vi "recondense_Splitt_Cluster.vi"(0 "Recondense-Monitor":T3 {"He3-Pot Heater %" format="%#_4g"; "He3-Pot Setpoint" format="%#_4g"; "Sorb Heater %" format="%#_4g"; "Sorb Setpoint" format="%#_4g"; "He3 Temp2" format="%#_4g"; "He3 Temp 1" format="%#_4g"; "1K Temp" format="%#_4g"; "Sorb Temp" format="%#_4g"}) -> (1 "Recondense-Status":T2, 2 "Recondense-Control":T1)   [LabVIEW 2019]
uses:
  Brosowski/BorowskiMonitor.ctl
  Brosowski/Borowski-Status-Cluster.ctl
  Brosowski/Borowski-Control-Cluster.ctl
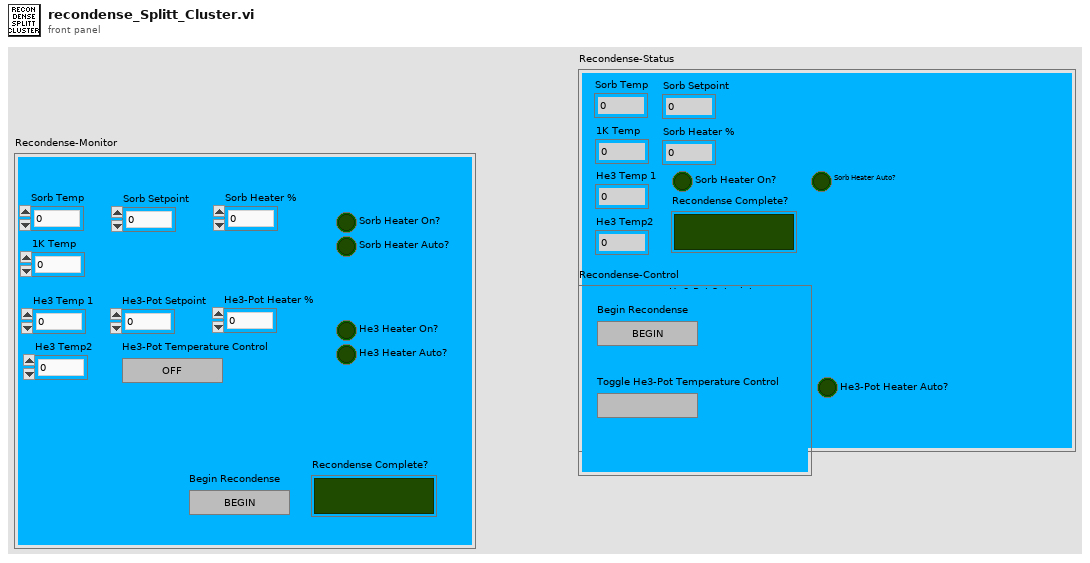
[diagram p1: front panel]
types:
  T1 = typedef "Borowski-Control-Cluster.ctl" = cluster{"Begin Recondense":bool, "Toggle He3-Pot Temperature Control":bool}
  T2 = typedef "Borowski-Status-Cluster.ctl" = cluster{"Sorb Temp":dbl, "1K Temp":dbl, "He3 Temp 1":dbl, "He3 Temp2":dbl, "Recondense Complete?":bool, "Sorb Heater Auto?":bool, "Sorb Heater On?":bool, "Sorb Setpoint":dbl, "Sorb Heater %":dbl, "He3-Pot Heater Auto?":bool, "He3-Pot Heater On?":bool, "He3-Pot Setpoint":dbl, "He3-Pot Heater %":dbl}
  T3 = typedef "BorowskiMonitor.ctl" = cluster{"Sorb Temp":dbl, "1K Temp":dbl, "He3 Temp 1":dbl, "He3 Temp2":dbl, "Recondense Complete?":bool, "Sorb Heater Auto?":bool, "Sorb Heater On?":bool, "Sorb Setpoint":dbl, "Sorb Heater %":dbl, "Begin Recondense":bool, "He3-Pot Setpoint":dbl, "He3-Pot Heater %":dbl, "He3 Heater Auto?":bool, "He3 Heater On?":bool, "He3-Pot Temperature Control":bool}
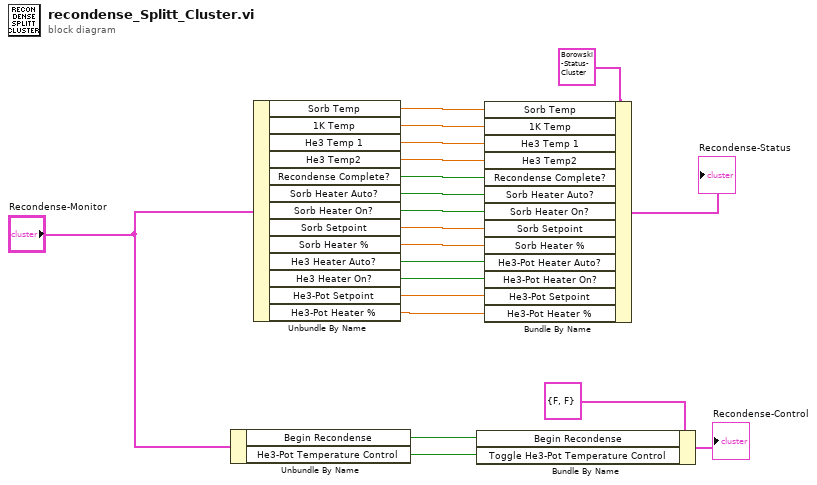
[diagram p0: block diagram]
diagram:
  n1 = Unbundle By Name("Recondense-Monitor") -> ("Begin Recondense"=w6:bool, "He3-Pot Temperature Control"=w5:bool)
  n2 = Unbundle By Name("Recondense-Monitor") -> ("Sorb Temp"=w18:dbl, "1K Temp"=w17:dbl, "He3 Temp 1"=w16:dbl, "He3 Temp2"=w15:dbl, "Recondense Complete?"=w14:bool, "Sorb Heater Auto?"=w13:bool, "Sorb Heater On?"=w12:bool, "Sorb Setpoint"=w11:dbl, "Sorb Heater %"=w10:dbl, "He3 Heater Auto?"=w1:bool, "He3 Heater On?"=w2:bool, "He3-Pot Setpoint"=w3:dbl, "He3-Pot Heater %"=w4:dbl)
  n3 = Bundle By Name(cluster=T1 {"Begin Recondense"=FALSE, "Toggle He3-Pot Temperature Control"=FALSE} ("Recondense-Control"), "Begin Recondense"=w6, "Toggle He3-Pot Temperature Control"=w5) -> (→"Recondense-Control":T1)
  n4 = Bundle By Name(cluster=T2 {"Sorb Temp"=0.0, "1K Temp"=0.0, "He3 Temp 1"=0.0, "He3 Temp2"=0.0, "Recondense Complete?"=FALSE, "Sorb Heater Auto?"=FALSE, "Sorb Heater On?"=FALSE, "Sorb Setpoint"=0.0, "Sorb Heater %"=0.0, "He3-Pot Heater Auto?"=FALSE, "He3-Pot Heater On?"=FALSE, "He3-Pot Setpoint"=0.0, "He3-Pot Heater %"=0.0} ("Recondense-Status"), "Sorb Temp"=w18, "1K Temp"=w17, "He3 Temp 1"=w16, "He3 Temp2"=w15, "Recondense Complete?"=w14, "Sorb Heater Auto?"=w13, "Sorb Heater On?"=w12, "Sorb Setpoint"=w11, "Sorb Heater %"=w10, "He3-Pot Heater Auto?"=w1, "He3-Pot Heater On?"=w2, "He3-Pot Setpoint"=w3, "He3-Pot Heater %"=w4) -> (→"Recondense-Status":T2)
